vi "RTD转换.vi"() -> ()   [LabVIEW 2018]
uses:
  <vilib>/Utility/TradDaqScaling.llb/Convert RTD Reading (scaler).vi
panel:
  in  "停止":bool
  out "温度计":dbl(slide) scale=0.0..100.0
  in  "输入电压":dbl
  in  "方程系数B":sgl=-5.80195e-07 caption="B" format="%0.5e"
  in  "方程系数A":sgl=0.00390802 caption="A" format="%0.5e"
  in  "激励电流":sgl=0.00015 caption="Iex" format="%0.3e"
  in  "0℃时电阻":sgl=100.0 caption="Ro" format="%0.2f"
  out "字符串":string="RTD转换；\n将RTD（电阻式温度传感器）读取得电压值转换为摄氏温度值"
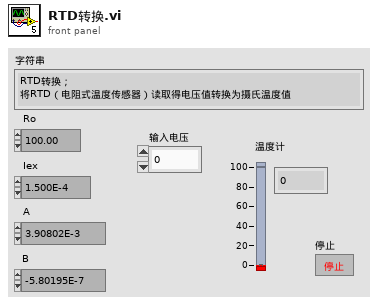
[diagram p1: front panel]
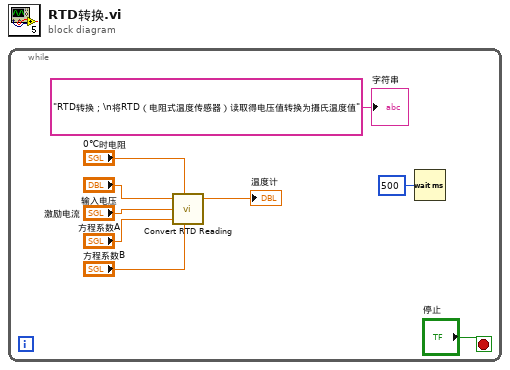
[diagram p0: block diagram]
diagram:
  n1 = while {
    stop <- "停止" stop-if-true
    n2 = call-poly <vilib>:"Convert RTD Reading.vi"("RTDvolts"="输入电压", "Ro"="0℃时电阻", "Iex"="激励电流", "A"="方程系数A", "B"="方程系数B") -> ("RTDtemp"=→"温度计":sgl)  [unwired: 2 in]
    n3 = Wait (ms)(milliseconds to wait=u32 500 ("等待时间（毫秒）")) -> ()  [unwired: 1 out]
    "字符串" <- "RTD转换；\n将RTD（电阻式温度传感器）读取得电压值转换为摄氏温度值"
  }
